vi "gm_measuringmode_flushing.vi"(9 "rt_vars in":T2, 10 "Output - Cluster gas in":T1 {"GM TS-2[°C]" format="%.2g"; "GM TS-1 [°C]" format="%.2g"; "GM DS-1 [bar]" format="%.4g"; "GM DS-2 [bar]" format="%.4g"; "GA1 h2 [%]" format="%.2g"; "GA1 co2 [%]" format="%.2g"; "GA1 ch4 [%]" format="%.2g"}, 11 "Input - Cluster gas in":T3) -> (1 "rt_vars out":T2, 2 "Output - Cluster gas out":T1 {"GM TS-2[°C]" format="%.2g"; "GM TS-1 [°C]" format="%.2g"; "GM DS-1 [bar]" format="%.4g"; "GM DS-2 [bar]" format="%.4g"; "GA1 h2 [%]" format="%.2g"; "GA1 co2 [%]" format="%.2g"; "GA1 ch4 [%]" format="%.2g"}, 3 "Input - Cluster gas out":T3)   [LabVIEW 2011]
uses:
  Input - Cluster gas.ctl
  Output - Cluster gas.ctl
panel:
  # "converted bool array!"
  # "mode :\n0: nothing\n1: quality\n2: quantity\n3: quality and quantity"
  # "converted bool array!"
  # "mode :\n0: nothing\n1: quality\n2: quantity\n3: quality and quantity"
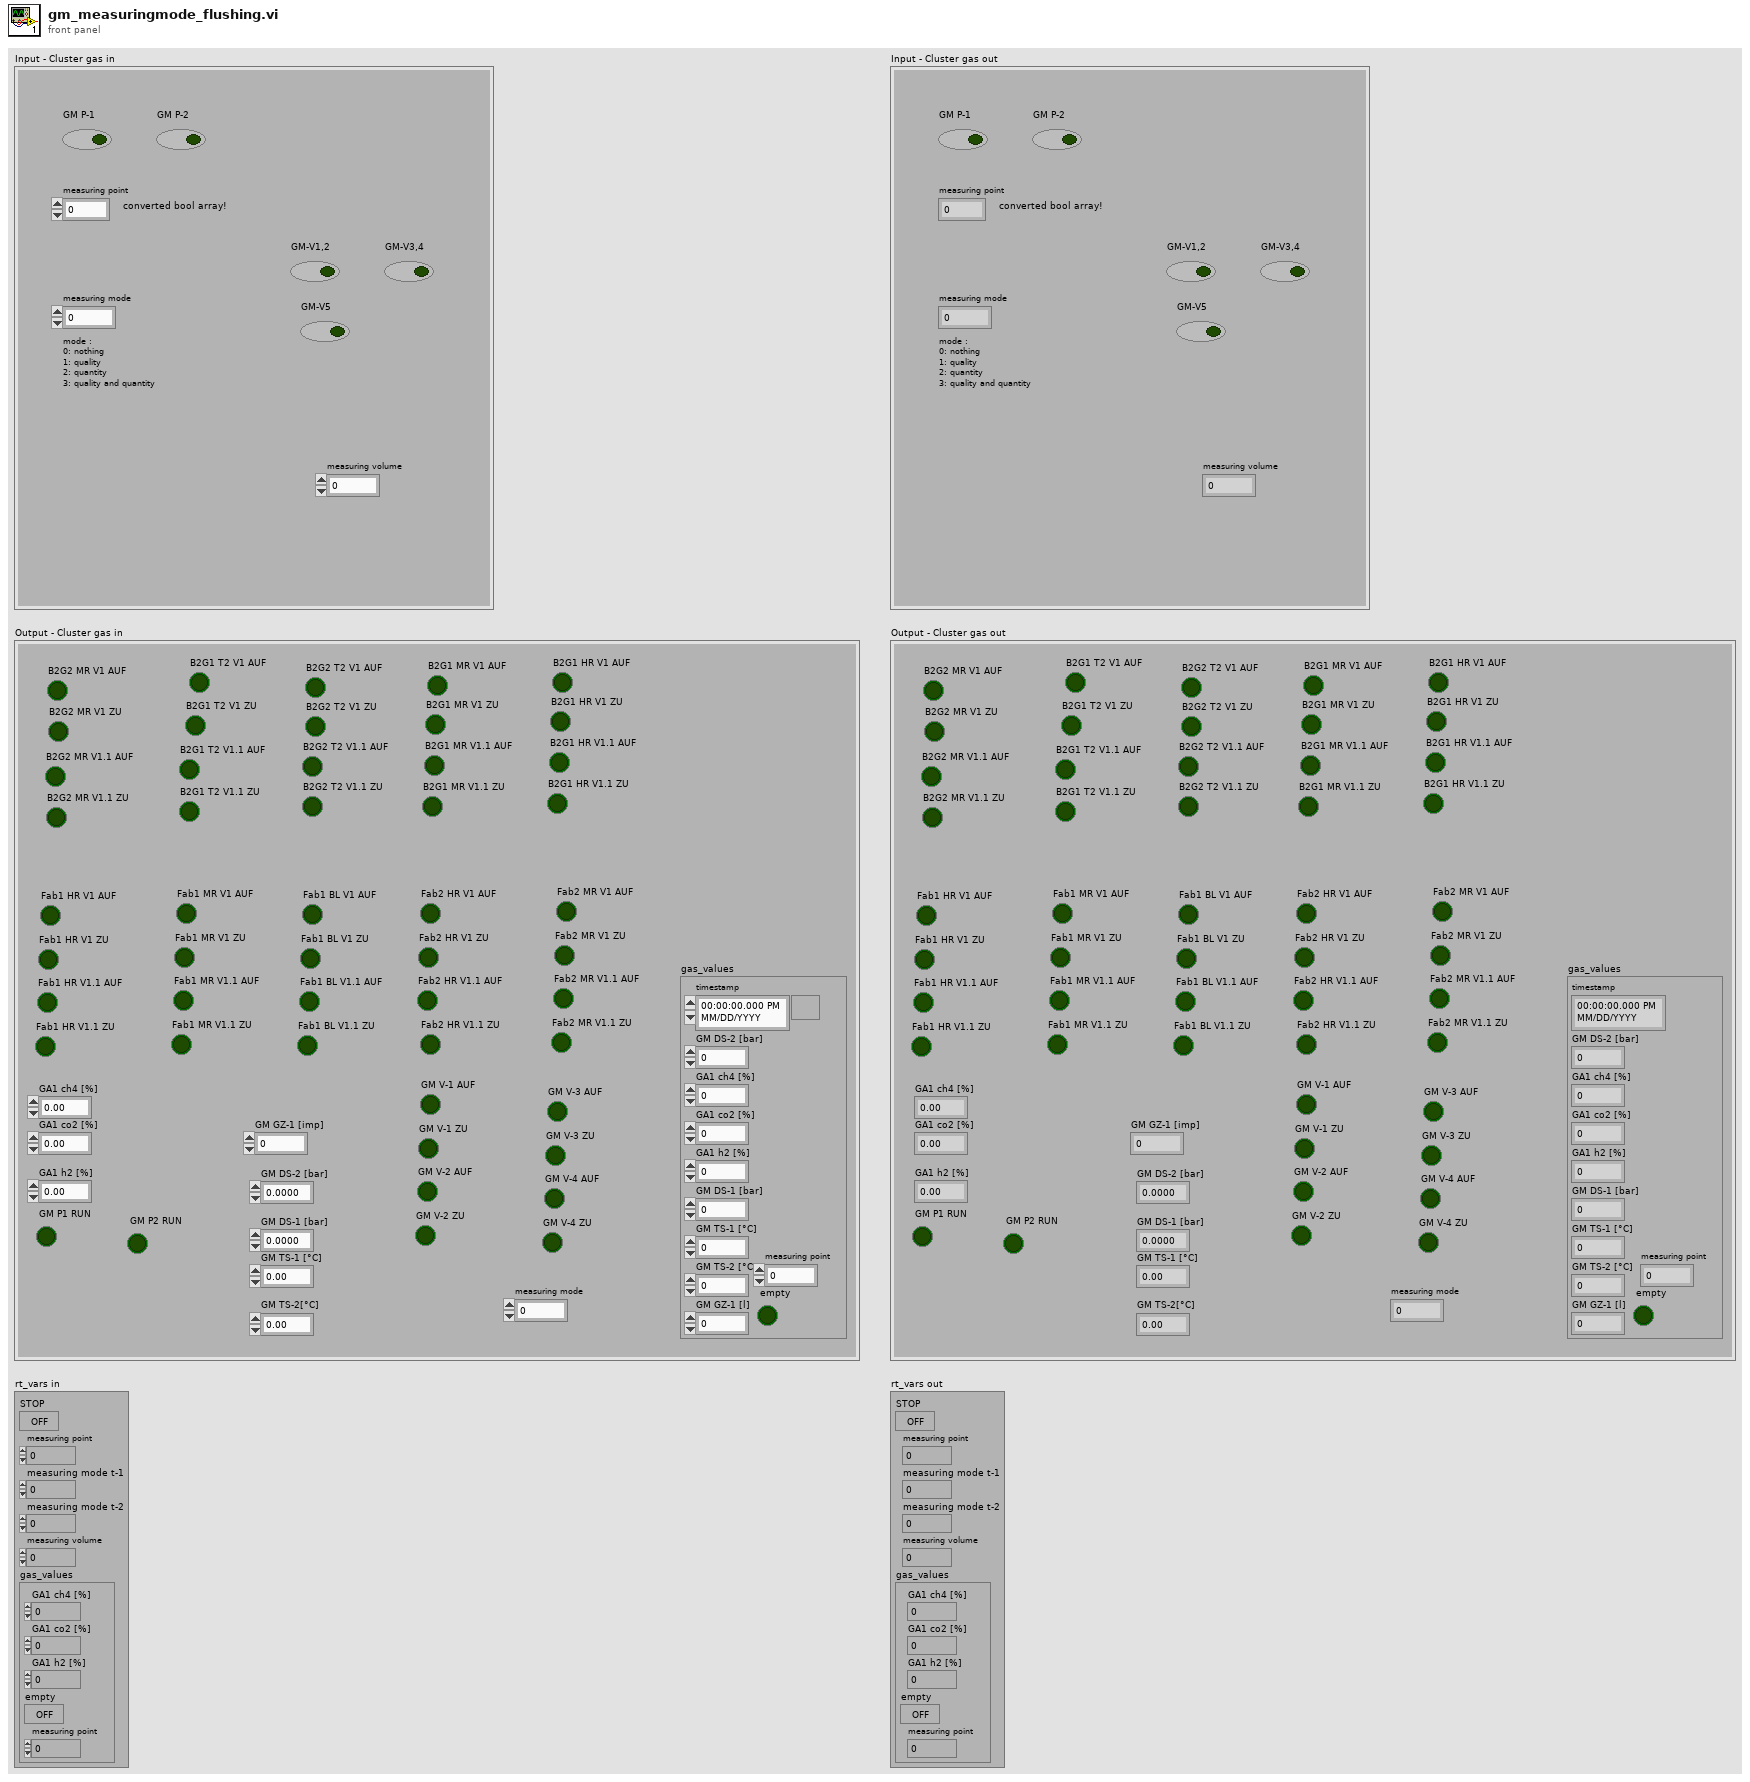
[diagram p1: front panel]
types:
  T1 = typedef "Output - Cluster gas.ctl" = cluster{"B2G2 MR V1.1 AUF":bool, "B2G2 MR V1.1 ZU":bool, "B2G2 MR V1 AUF":bool, "B2G2 MR V1 ZU":bool, "B2G1 T2 V1 AUF":bool, "B2G1 T2 V1 ZU":bool, "B2G1 T2 V1.1 AUF":bool, "B2G1 T2 V1.1 ZU":bool, "B2G2 T2 V1 AUF":bool, "B2G2 T2 V1 ZU":bool, "B2G2 T2 V1.1 ZU":bool, "B2G2 T2 V1.1 AUF":bool, "B2G1 MR V1 AUF":bool, "B2G1 MR V1 ZU":bool, "B2G1 MR V1.1 AUF":bool, "B2G1 MR V1.1 ZU":bool, "B2G1 HR V1 AUF":bool, "B2G1 HR V1 ZU":bool, "B2G1 HR V1.1 AUF":bool, "B2G1 HR V1.1 ZU":bool, "Fab1 HR V1 AUF":bool, "Fab1 HR V1 ZU":bool, "Fab1 HR V1.1 AUF":bool, "Fab1 HR V1.1 ZU":bool, "Fab1 MR V1 AUF":bool, "Fab1 MR V1 ZU":bool, "Fab1 MR V1.1 AUF":bool, "Fab1 MR V1.1 ZU":bool, "Fab1 BL V1 AUF":bool, "Fab1 BL V1 ZU":bool, "Fab1 BL V1.1 AUF":bool, "Fab1 BL V1.1 ZU":bool, "Fab2 HR V1 AUF":bool, "Fab2 HR V1 ZU":bool, "Fab2 HR V1.1 AUF":bool, "Fab2 HR V1.1 ZU":bool, "Fab2 MR V1 AUF":bool, "Fab2 MR V1 ZU":bool, "Fab2 MR V1.1 AUF":bool, "Fab2 MR V1.1 ZU":bool, "GA1 ch4 [%]":dbl, "GA1 co2 [%]":dbl, "GA1 h2 [%]":dbl, "GM P1 RUN":bool, "GM V-1 AUF":bool, "GM V-1 ZU":bool, "GM V-2 AUF":bool, "GM V-2 ZU":bool, "GM V-3 AUF":bool, "GM V-3 ZU":bool, "GM V-4 AUF":bool, "GM V-4 ZU":bool, "GM P2 RUN":bool, "GM GZ-1 [imp]":u32, "GM DS-2 [bar]":dbl, "GM DS-1 [bar]":dbl, "GM TS-1 [°C]":dbl, "GM TS-2[°C]":dbl, "gas_values":cluster{"timestamp":timestamp, "GM DS-2 [bar]":dbl, "GA1 ch4 [%]":dbl, "GA1 co2 [%]":dbl, "GA1 h2 [%]":dbl, "GM DS-1 [bar]":dbl, "GM TS-1 [°C]":dbl, "GM TS-2 [°C]":dbl, "GM GZ-1 [l]":dbl, "empty":bool, "measuring point":u8}, "measuring mode":u8}
  T2 = cluster{"STOP":bool, "measuring point":u32, "measuring mode t-1":u8, "measuring mode t-2":u8, "measuring volume":u32, "gas_values":cluster{"GA1 ch4 [%]":dbl, "GA1 co2 [%]":dbl, "GA1 h2 [%]":dbl, "empty":bool, "measuring point":u8}}
  T3 = typedef "Input - Cluster gas.ctl" = cluster{"GM P-1":bool, "GM P-2":bool, "measuring point":u32, "measuring mode":u8, "GM-V1,2":bool, "GM-V3,4":bool, "GM-V5":bool, "measuring volume":u32}
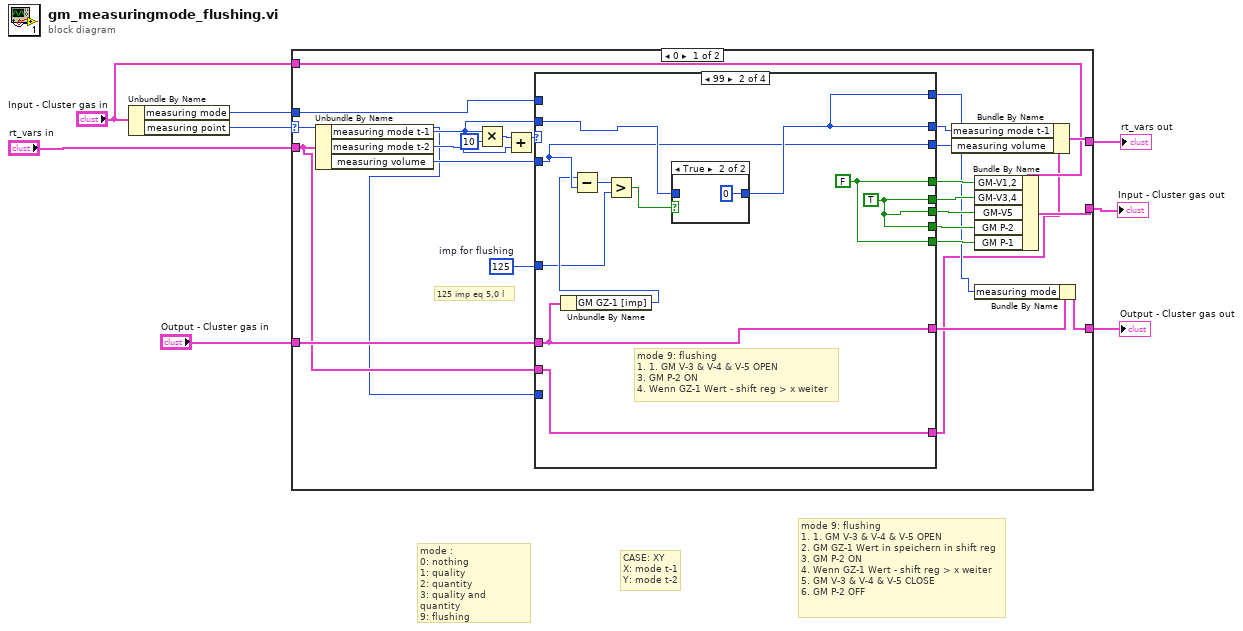
[diagram p0: block diagram]
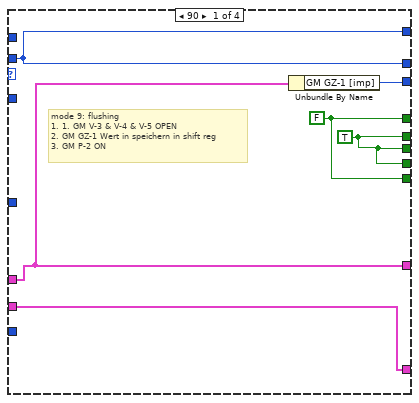
[diagram p2: hidden frame]
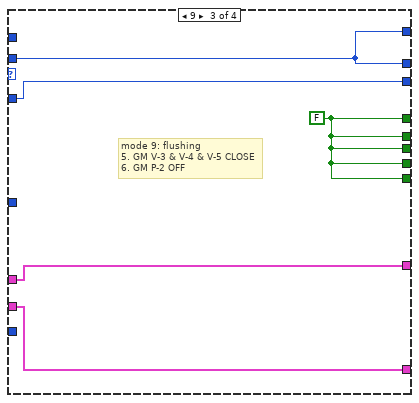
[diagram p4: hidden frame]
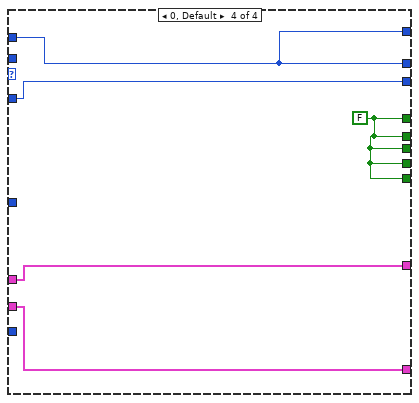
[diagram p5: hidden frame]
diagram:
  # "mode :\n0: nothing\n1: quality\n2: quantity\n3: quality and quantity\n9: flushing"
  # "mode 9: flushing\n1. 1. GM V-3 & V-4 & V-5 OPEN\n2. GM GZ-1 Wert in speichern in shift reg\n3. GM P-2 ON\n4. Wenn GZ-1 Wert - shift reg > x weiter \n5. GM V-3 & V-4 & V-5 CLOSE\n6. GM P-2 OFF"
  # "CASE: XY\nX: mode t-1\nY: mode t-2"
  n1 = Unbundle By Name("Input - Cluster gas in") -> ("measuring mode"=w2:u8, "measuring point"=w1:u32)
  n2 = case shown="0" w1 {
    selector: w1 -> [w9 _]
    tunnel: w2 -> [w33 _]
    tunnel: "Output - Cluster gas in" -> [w29 w65]
    tunnel: [w14 w65] -> w4
    tunnel: "rt_vars in" -> [w12 w64]
    tunnel: [w25 w64] -> w6
    tunnel: "Input - Cluster gas in" -> [w17 w63]
    tunnel: [w16 w63] -> w8
    frame 0 {
      w10 = u32 125  # imp for flushing
      # "125 imp eq 5,0 l"
      n3 = Unbundle By Name(w12) -> ("measuring mode t-1"=w28:u8, "measuring mode t-2"=w27:u8, "measuring volume"=w26:u32)
      n4 = Multiply(x=w28, y=u8 10) -> (x*y=w32:u8)
      n5 = Add(x=w32, y=w27) -> (x+y=w31:u8)
      n6 = case shown="99" w31 {
        tunnel: w33 -> [_ _ _ w62]
        tunnel: [w38 w49 w56 w62] -> w24
        tunnel: [w39 w41 w57 w61] -> w22
        tunnel: [w34 w40 w57 w61] -> w21
        tunnel: [w34 w40 w57 w61] -> w20
        tunnel: [w38 w49 w56 w62] -> w13
        tunnel: [w36 w48 w55 w58] -> w23
        tunnel: [w34 w40 w57 w61] -> w19
        tunnel: [w39 w41 w57 w61] -> w18
        tunnel: w26 -> [_ w48 w55 w58]
        tunnel: w28 -> [w38 w50 w56 _]
        tunnel: w29 -> [w37 w46 w53 w60]
        tunnel: [w37 w46 w53 w60] -> w15
        tunnel: w9 -> [_ _ _ _]
        tunnel: w12 -> [w35 w44 w54 w59]
        tunnel: [w35 w44 w54 w59] -> w11
        tunnel: w10 -> [_ w43 _ _]
        frame 90 {
          w39 = FALSE ("GM-V3,4")
          w34 = TRUE ("GM-V3,4")
          # "mode 9: flushing\n1. 1. GM V-3 & V-4 & V-5 OPEN\n2. GM GZ-1 Wert in speichern in shift reg\n3. GM P-2 ON"
          n7 = Unbundle By Name(w37) -> ("GM GZ-1 [imp]"=w36:u32)
        }
        frame 99 {
          w41 = FALSE ("GM-V3,4")
          w40 = TRUE ("GM-V3,4")
          # "mode 9: flushing\n1. 1. GM V-3 & V-4 & V-5 OPEN\n3. GM P-2 ON\n4. Wenn GZ-1 Wert - shift reg > x weiter"
          n8 = Unbundle By Name(w46) -> ("GM GZ-1 [imp]"=w45:u32)
          n9 = Subtract(x=w45, y=w48) -> (x-y=w47:u32)
          n10 = Greater?(x=w47, y=w43) -> (0:w42:bool)
          n11 = case shown="True" w42 {
            tunnel: w50 -> [w51 _]
            tunnel: [w51 u8 0 ("measuring mode t-1")] -> w49
            frame False {
            }
            frame True {
            }
          }
        }
        frame 9 {
          w57 = FALSE ("GM-V3,4")
          # "mode 9: flushing\n5. GM V-3 & V-4 & V-5 CLOSE\n6. GM P-2 OFF"
        }
        frame 0, Default {
          w61 = FALSE ("GM-V3,4")
        }
      }
      n12 = Bundle By Name(cluster=w11, "measuring mode t-1"=w24, "measuring volume"=w23) -> (w25:T2)
      n13 = Bundle By Name(cluster=w17, "GM-V1,2"=w22, "GM-V3,4"=w21, "GM-V5"=w20, "GM P-2"=w19, "GM P-1"=w18) -> (w16:T3)
      n14 = Bundle By Name(cluster=w15, "measuring mode"=w13) -> (w14:T1)
    }
    frame 1, Default {
    }
  }
  "Input - Cluster gas out" <- w8
  "rt_vars out" <- w6
  "Output - Cluster gas out" <- w4
